vi "4-1 SoundVIEW.vi"() -> ()   [LabVIEW 2014]
doc: "------------------------------------\nAuther: Koji Ohashi\nModified: Hirotake Watashima\nCopyright (c) 2020 Japan LabVIEW Users Group, Volunteer members.\nThis VI is released under the MIT License.\nhttp://opensource.org/licenses/mit-license.php\n------------------------------------"
uses:
  4-1 subVI_SoundVIEW/svState.ctl
  <vilib>/sound2/lvsound2.llb/Sound Data Format.ctl
  <vilib>/sound2/lvsound2.llb/Sampling Mode.ctl
  <vilib>/sound2/lvsound2.llb/Sound Input Task ID.ctl
  4-1 subVI_SoundVIEW/dataInfo.ctl
  <vilib>/sound2/lvsound2.llb/Sound Input Read (DBL).vi
  <vilib>/sound2/lvsound2.llb/Sound Output Write (DBL Single).vi
panel:
  out "error out":errorcluster
  out "recLED":bool
  out "Spectrogram":dbl[][](graph)
  out "Waveform Graph":dbl[](graph)
  in  "Save As Button":bool
  in  "Open Button":bool
  in  "Play Button":bool
  in  "Stop Button":bool
  in  "Record Button":bool
  out "SoundViewState":T1=enum."idle"
  in  "stop":bool
  in  "Recording Time (5sec)":i32=5
  in  "Input Source":bool
  # "SoundVIEW"
  # "PC\nMic"
  # "PC : Record sound played on PC*\nMic : Built-in microphone"
  # "*Enable the stereo mixer in the recording tab of the sound control panel of Windows 10"
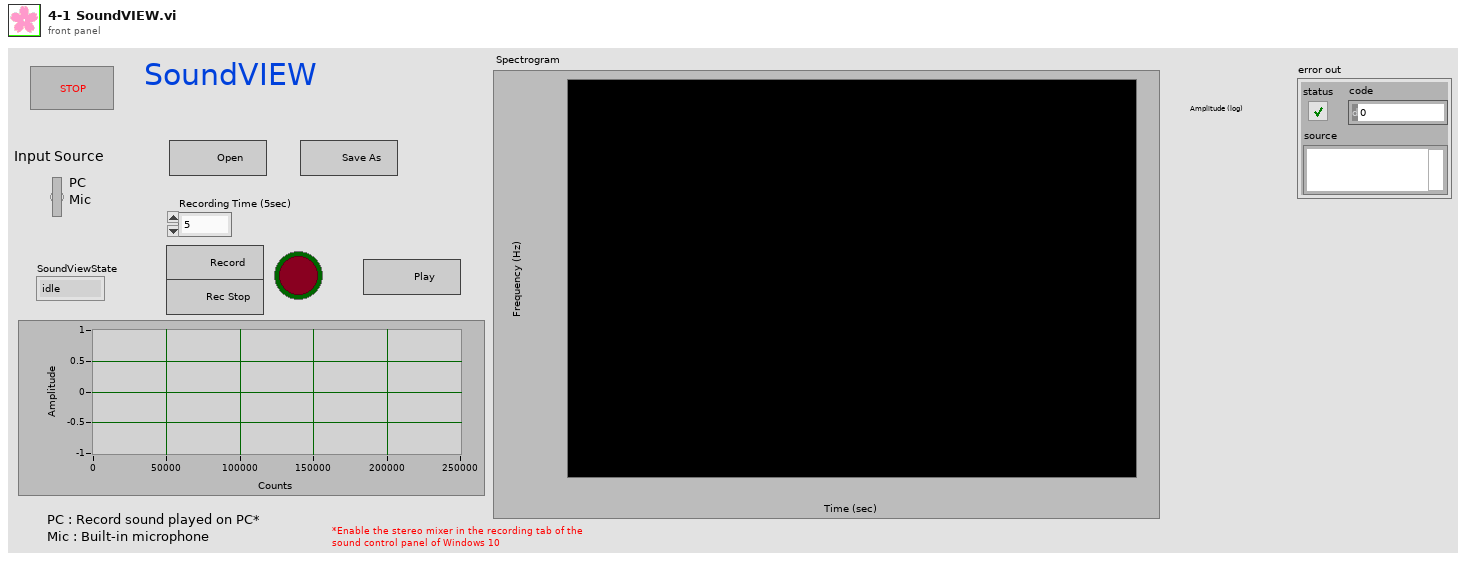
[diagram p1: front panel]
types:
  T1 = typedef "svState.ctl" = enum16{"initialize", "idle", "recStart", "Recording", "recStop", "Play", "Save", "Load"}
  T2 = typedef "dataInfo.ctl" = cluster{"task ID":T3, "Sound":T4, "DataCounts":i32, "blockCounts":i32, "Data":dbl[]}
  T3 = typedef "Sound Input Task ID.ctl" = u32
  T4 = typedef "Sound Data Format.ctl" = cluster{"sample rate (S/s)":dbl, "number of channels":i32, "bits per sample":i32}
  T5 = typedef "Sampling Mode.ctl" = i32
  T6 = typedef "Sound Output Task ID.ctl" = u32
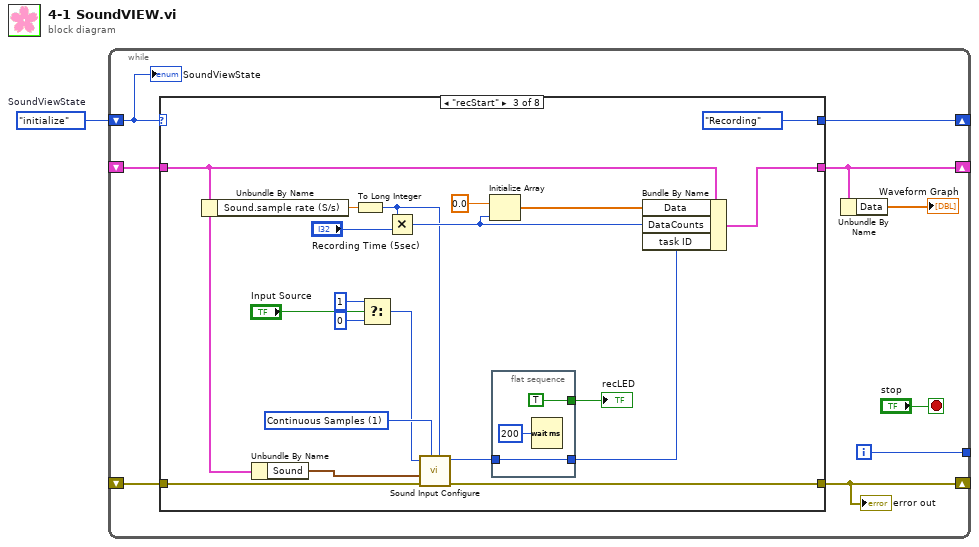
[diagram p0: block diagram]
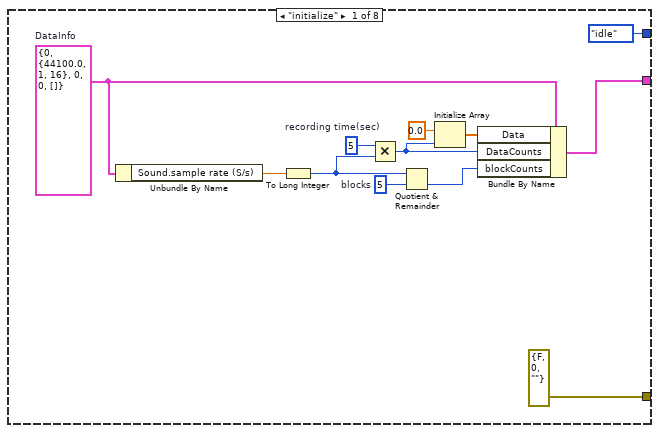
[diagram p2: hidden frame]
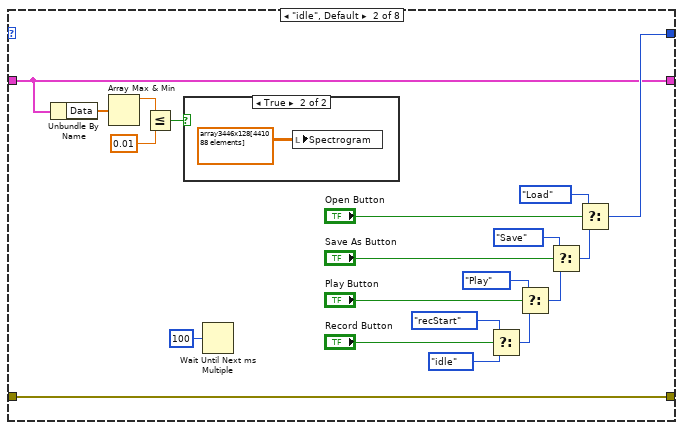
[diagram p3: hidden frame]
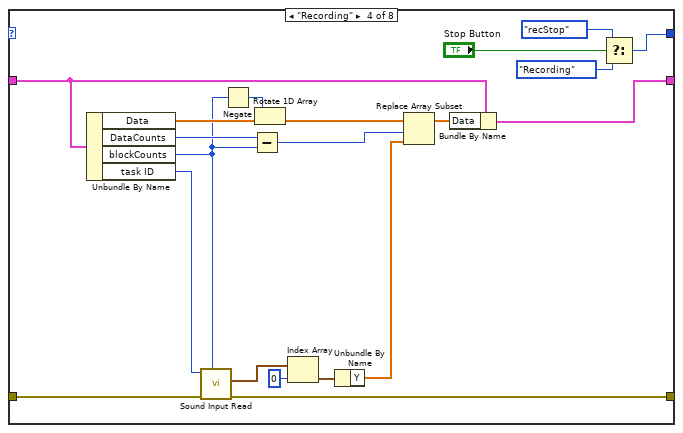
[diagram p5: hidden frame]
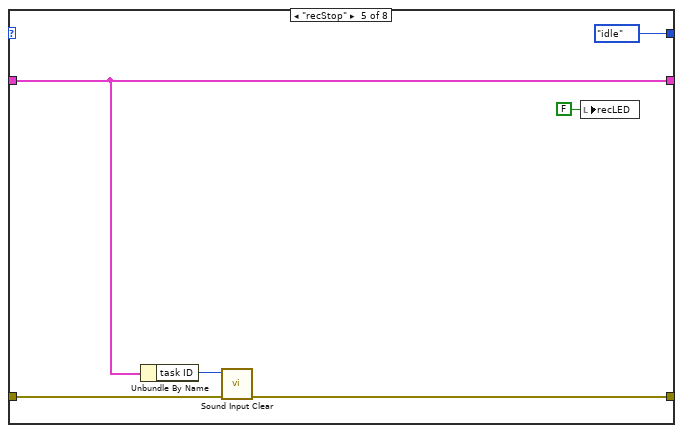
[diagram p6: hidden frame]
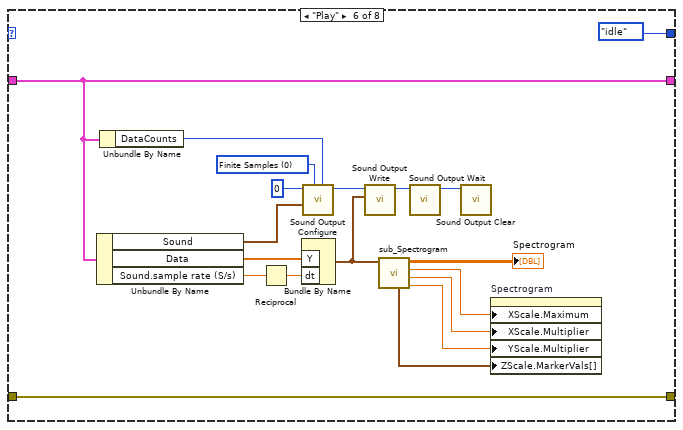
[diagram p7: hidden frame]
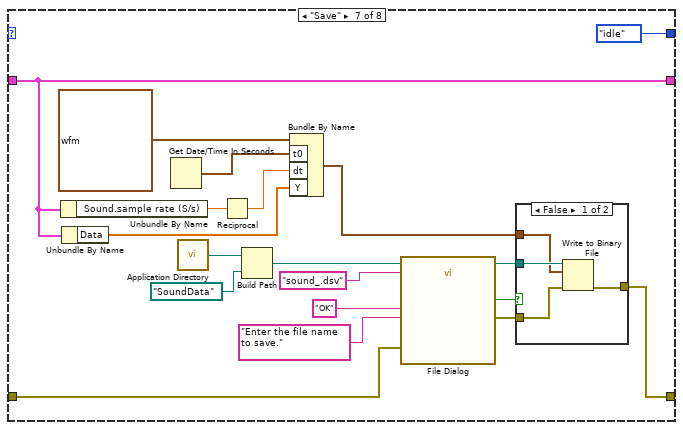
[diagram p8: hidden frame]
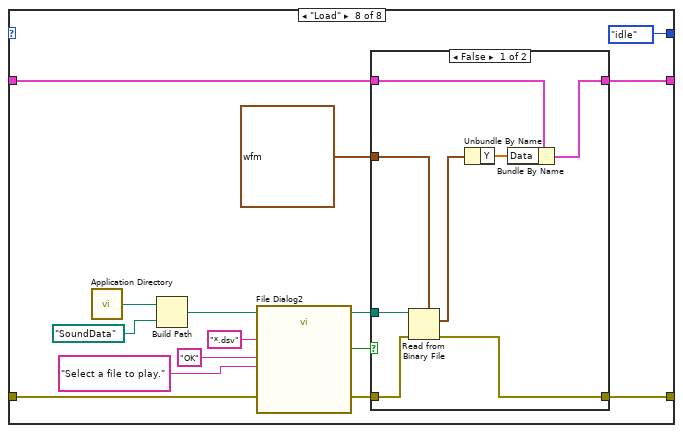
[diagram p10: hidden frame]
diagram:
  w1 = svState."initialize"  # SoundViewState
  n1 = while {
    shift-right: [w8] -> _
    shift-left: w1 -> [w9]
    shift-right: [w6] -> _
    shift-left: _ -> [w7]
    shift-right: [w4] -> _
    shift-left: _ -> [w5]
    tunnel: [w2] -> _
    i -> [w2]
    stop <- "stop" stop-if-true
    n2 = case shown="\"recStart\"" w9 {
      tunnel: [svState."idle" ("SoundViewState") w28 svState."Recording" ("SoundViewState") w74 svState."idle" ("SoundViewState") svState."idle" ("SoundViewState") svState."idle" ("SoundViewState") svState."idle" ("SoundViewState")] -> w8
      tunnel: w7 -> [_ w38 w58 w85 w90 w110 w120 w144]
      tunnel: [errorcluster {"status"=FALSE, "code"=0, "source"=""} ("error in (no error)") w38 w44 w86 w91 w110 w121 w145] -> w6
      tunnel: [w12 w24 w54 w70 w88 w99 w113 w136] -> w4
      tunnel: w5 -> [_ w24 w52 w71 w88 w99 w113 w137]
      frame "initialize" {
        w21 = 5  # recording time(sec)
        w20 = 5  # blocks
        w13 = T2 {"task ID"=0, "Sound"={"sample rate (S/s)"=44100.0, "number of channels"=1, "bits per sample"=16}, "DataCounts"=0, "blockCounts"=0, "Data"=[]}  # DataInfo
        n3 = Unbundle By Name(w13) -> ("Sound.sample rate (S/s)"=w18:dbl)
        n4 = To Long Integer(number=w18) -> (32bit integer=w16:i32)
        n5 = Multiply(x=w21, y=w16) -> (x*y=w15:i32)
        n6 = Quotient & Remainder(x=w16, y=w20) -> (floor(x/y)=w14:i32)  [unwired: 1 out]
        n7 = Initialize Array(0.0 ("element"), w15) -> (w17:dbl[])
        n8 = Bundle By Name(cluster=w13, "Data"=w17, "DataCounts"=w15, "blockCounts"=w14) -> (w12:T2)
      }
      frame "idle", Default {
        n9 = Unbundle By Name(w24) -> ("Data"=w23:dbl[])
        n10 = Array Max & Min(array=w23) -> (max value=w27:dbl)  [unwired: 3 out]
        n11 = Less Or Equal?(x=w27, y=0.01) -> (x <= y?=w25:bool)
        n12 = case shown="TRUE" w25 {
          frame False {
          }
          frame True {
            n13 = local write "Spectrogram"(dbl[][] array3446x128[441088 elements] ("Array")) -> ()
          }
        }
        n14 = Wait Until Next ms Multiple(millisecond multiple=u32 100) -> ()  [unwired: 1 out]
        n15 = Select(t=svState."recStart" ("SoundViewState"), s="Record Button", f=svState."idle" ("SoundViewState")) -> (s? t:f=w36:T1)
        n16 = Select(t=svState."Play" ("SoundViewState"), s="Play Button", f=w36) -> (s? t:f=w32:T1)
        n17 = Select(t=svState."Save" ("SoundViewState"), s="Save As Button", f=w32) -> (s? t:f=w29:T1)
        n18 = Select(t=svState."Load" ("SoundViewState"), s="Open Button", f=w29) -> (s? t:f=w28:T1)
      }
      frame "recStart" {
        w59 = T5 1 items=["Finite Samples", "Continuous Samples"] ("sample mode")
        n19 = Unbundle By Name(w52) -> ("Sound.sample rate (S/s)"=w50:dbl)
        n20 = Unbundle By Name(w52) -> ("Sound"=w53:T4)
        n21 = To Long Integer(number=w50) -> (32bit integer=w46:i32)
        n22 = Select(t=u32 1, s="Input Source", f=u32 0) -> (s? t:f=w49:u32)
        n23 = Multiply(x=w46, y="Recording Time (5sec)") -> (x*y=w47:i32)
        n24 = call <vilib>:"Sound Input Configure.vi"("number of samples/ch"=w46, "sample mode"=w59, "error in (no error)"=w58, "sound format"=w53, "device ID"=w49) -> ("error out"=w44:errorcluster, "task ID"=w45:T3)  [unwired: 5 in]
        n25 = Initialize Array(0.0 ("element"), w47) -> (w55:dbl[])
        n26 = flat-sequence {
          tunnel: [TRUE ("recLED")] -> w56
          tunnel: [w64] -> w48
          tunnel: w45 -> [w64]
          frame #0 {
            n27 = Wait (ms)(milliseconds to wait=u32 200) -> ()  [unwired: 1 out]
          }
        }
        n28 = Bundle By Name(cluster=w52, "Data"=w55, "DataCounts"=w47, "task ID"=w48) -> (w54:T2)
        "recLED" <- w56
      }
      frame "Recording" {
        n29 = Unbundle By Name(w71) -> ("Data"=w73:dbl[], "DataCounts"=w69:i32, "blockCounts"=w68:i32, "task ID"=w67:T3)
        n30 = call-poly <vilib>:"Sound Input Read.vi"("number of samples/ch"=w68, "error in (no error)"=w85, "task ID"=w67) -> ("error out"=w86:errorcluster, "data"=w80:waveform(dbl)[])  [unwired: 6 in, 1 out]
        n31 = Negate(x=w68) -> (-x=w84:i32)
        n32 = Subtract(x=w69, y=w68) -> (x-y=w77:i32)
        n33 = Rotate 1D Array(1:w73, 2:w84) -> (0:w78:dbl[])
        n34 = Index Array(array=w80, index=0) -> (element=w79:waveform(dbl))
        n35 = Unbundle By Name(w79) -> ("Y"=w76:dbl[])
        n36 = Replace Array Subset(array=w78, new element=w76, index=w77) -> (w72:dbl[])
        n37 = Bundle By Name(cluster=w71, "Data"=w72) -> (w70:T2)
        n38 = Select(t=svState."recStop" ("SoundViewState"), s="Stop Button", f=svState."Recording" ("SoundViewState")) -> (s? t:f=w74:T1)
      }
      frame "recStop" {
        n39 = Unbundle By Name(w88) -> ("task ID"=w87:T3)
        n40 = call <vilib>:"Sound Input Clear.vi"("error in (no error)"=w90, "task ID"=w87) -> ("error out"=w91:errorcluster)  [unwired: 9 in]
        n41 = local write "recLED"(FALSE ("recLED")) -> ()
      }
      frame "Play" {
        w108 = T5 0 items=["Finite Samples", "Continuous Samples"] ("sample mode")
        n42 = Unbundle By Name(w99) -> ("Sound"=w97:T4, "Data"=w98:dbl[], "Sound.sample rate (S/s)"=w106:dbl)
        n43 = Unbundle By Name(w99) -> ("DataCounts"=w100:i32)
        n44 = Reciprocal(x=w106) -> (1/x=w105:dbl)
        n45 = Bundle By Name("Y"=w98, "dt"=w105) -> (w102:waveform(dbl))  [unwired: 1 in]
        n46 = call <vilib>:"Sound Output Configure.vi"("number of samples/ch"=w100, "sample mode"=w108, "sound format"=w97, "device ID"=u32 0) -> ("task ID"=w107:T6)  [unwired: 6 in, 1 out]
        n47 = call-poly <vilib>:"Sound Output Write.vi"("data"=w102, "task ID"=w107) -> ("task ID out"=w104:T6)  [unwired: 8 in, 1 out]
        n48 = call "sub_Spectrogram.vi"("data"=w102) -> ("Y Scale.Offset and Multiplier:Multiplier"=w93:dbl, "X Scale.Offset and Multiplier:Multiplier"=w94:dbl, "X Scale.Range:Maximum"=w95:dbl, "STFT Spectrogram"=→"Spectrogram":dbl[][], "Z Scale.Marker Values[]"=w96:cluster{dbl, u32}[])  [unwired: 6 in]
        n49 = call <vilib>:"Sound Output Wait.vi"("task ID"=w104) -> ("task ID out"=w103:T6)  [unwired: 9 in, 1 out]
        n50 = call <vilib>:"Sound Output Clear.vi"("task ID"=w103) -> ()  [unwired: 10 in, 1 out]
        n51 = property on="Spectrogram" class="IntGraph (指定)"("XScale.Maximum"=w95, "XScale.Multiplier"=w94, "YScale.Multiplier"=w93, "ZScale.MarkerVals[]"=w96) -> ()  [unwired: 2 in, 2 out]
      }
      frame "Save" {
        n52 = Unbundle By Name(w113) -> ("Sound.sample rate (S/s)"=w128:dbl)
        n53 = Unbundle By Name(w113) -> ("Data"=w112:dbl[])
        n54 = Get Date/Time In Seconds() -> (seconds since 1Jan1904=w118:timestamp)
        n55 = call <vilib>:"Application Directory.vi"() -> ("Application Directory"=w117:path)
        n56 = Reciprocal(x=w128) -> (1/x=w127:dbl)
        n57 = Build Path(base path=w117, name or relative path=path "SoundData") -> (appended path=w116:path)
        n58 = Bundle By Name(cluster=waveform(dbl) {"t0"=timestamp(0 s since 1904-01-01), "dt"=1.0, "Y"=[]} ("Waveform"), "t0"=w118, "dt"=w127, "Y"=w112) -> (w114:waveform(dbl))
        n59 = call "File Dialog"("start path"=w116, "prompt"="Enter the file name to save.", "button label"="OK", "default name"="sound_.dsv", "error in"=w120) -> ("selected path"=w123:path, "cancelled"=w119:bool, "error out"=w122:errorcluster)  [unwired: 7 in, 1 out]
        n60 = case shown="FALSE" w119 {
          tunnel: w123 -> [w134 _]
          tunnel: w122 -> [w132 w135]
          tunnel: [w133 w135] -> w121
          tunnel: w114 -> [w131 _]
          frame False {
            n61 = Write to Binary File(file (use dialog)=w134, data=w131, error in=w132) -> (error out=w133:errorcluster)  [unwired: 3 in, 2 out]
          }
          frame True {
          }
        }
      }
      frame "Load" {
        n62 = call <vilib>:"Application Directory.vi"() -> ("Application Directory"=w140:path)
        n63 = Build Path(base path=w140, name or relative path=path "SoundData") -> (appended path=w138:path)
        n64 = call "File Dialog2"("start path"=w138, "prompt"="Select a file to play.", "button label"="OK", "error in"=w144, "pattern (all files)"="*.dsv") -> ("selected path"=w147:path, "cancelled"=w148:bool, "error out"=w146:errorcluster)  [unwired: 7 in, 1 out]
        n65 = case shown="FALSE" w148 {
          tunnel: w147 -> [w158 _]
          tunnel: w146 -> [w155 w160]
          tunnel: [w154 w160] -> w145
          tunnel: waveform(dbl) {"t0"=timestamp(0 s since 1904-01-01), "dt"=1.0, "Y"=[]} ("Waveform") -> [w157 _]
          tunnel: w137 -> [w153 w159]
          tunnel: [w151 w159] -> w136
          frame False {
            n66 = Read from Binary File(5:w157, 8:w155, 11:w158) -> (0:w154:errorcluster, 2:w156:waveform(dbl))  [unwired: 3 in, 2 out]
            n67 = Unbundle By Name(w156) -> ("Y"=w152:dbl[])
            n68 = Bundle By Name(cluster=w153, "Data"=w152) -> (w151:T2)
          }
          frame True {
          }
        }
      }
    }
    "error out" <- w6
    n69 = Unbundle By Name(w4) -> ("Data"=→"Waveform Graph":dbl[])
    "SoundViewState" <- w9
  }
